vi "FPGA Rate.vi"(11 "FPGA Rate (kS/s)":sgl) -> (2 "FPGA Period (ms)":sgl, 3 "FPGA Period(us)":u32)   [LabVIEW 2018]
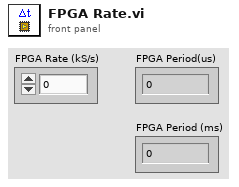
[diagram p1: front panel]
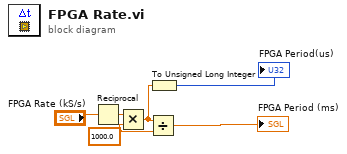
[diagram p0: block diagram]
diagram:
  w5 = sgl 1000.0 ("y")
  n1 = Reciprocal(x="FPGA Rate (kS/s)") -> (1/x=w1:sgl)
  n2 = Multiply(x=w1, y=w5) -> (x*y=w6:sgl)
  n3 = Divide(x=w6, y=w5) -> (x/y=→"FPGA Period (ms)":sgl)
  n4 = To Unsigned Long Integer(number=w6) -> (unsigned 32bit integer=→"FPGA Period(us)":u32)
